vi "Adjust GraphScale.vi"(11 "WaveformChart in":refnum<vi>) -> (3 "WaveformChart out":refnum<vi>)   [LabVIEW 2018]
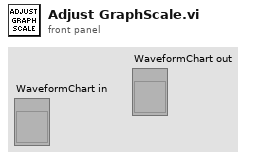
[diagram p1: front panel]
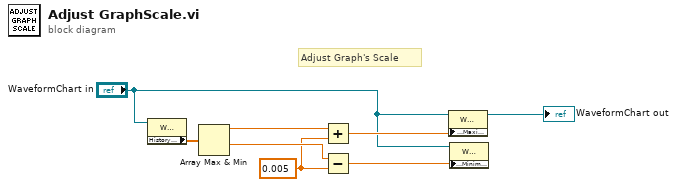
[diagram p0: block diagram]
diagram:
  w3 = 0.005 ("notification")
  # "Adjust Graph's Scale"
  n1 = property on="Property Node" class="WFChart (strict)"(reference="WaveformChart in") -> ("History Data"=w6:dbl[])  [unwired: 1 in, 2 out]
  n2 = Array Max & Min(array=w6) -> (max value=w7:dbl, min value=w8:dbl)  [unwired: 2 out]
  n3 = Add(x=w7, y=w3) -> (x+y=w4:dbl)
  n4 = Subtract(x=w8, y=w3) -> (x-y=w5:dbl)
  n5 = property on="Property Node" class="WFChart (strict)"(reference="WaveformChart in", "YScale.Maximum"=w4) -> (reference out=→"WaveformChart out":refnum<vi>)  [unwired: 1 in, 1 out]
  n6 = property on="Property Node" class="WFChart (strict)"(reference="WaveformChart in", "YScale.Minimum"=w5) -> ()  [unwired: 1 in, 2 out]
